vi "ContainsFile_WithFileIncluded_ReturnsTrue.vi"() -> ()   [LabVIEW 2019, in "WhitelistTest.lvlib"]
uses:
  WhitelistTest.lvlib
  Whitelist/Whitelist.lvclass
  Assertion/Assertion.lvlib
panel:
  out "error out":errorcluster
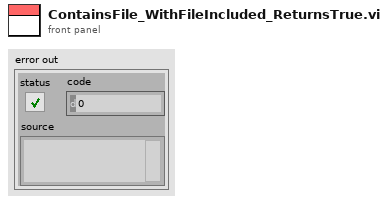
[diagram p1: front panel]
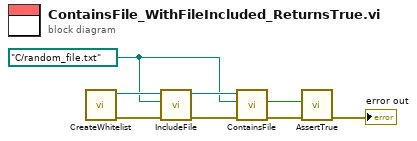
[diagram p0: block diagram]
diagram:
  w4 = path "C:/random_file.txt" ("Path")
  n1 = call "CreateWhitelist.vi"() -> ("error out"=w8:errorcluster, "Whitelist out"=w6:refnum<class "Whitelist.lvclass">)  [unwired: 10 in]
  n2 = call "IncludeFile.vi"("error in (no error)"=w8, "Path"=w4, "Whitelist in"=w6) -> ("error out"=w7:errorcluster, "Whitelist out"=w5:refnum<class "Whitelist.lvclass">)  [unwired: 7 in]
  n3 = call "ContainsFile.vi"("error in (no error)"=w7, "Path"=w4, "Whitelist in"=w5) -> ("error out"=w2:errorcluster, "Is Whitelisted?"=w3:bool)  [unwired: 6 in, 1 out]
  n4 = call "AssertTrue.vi"("error in (no error)"=w2, "Condition"=w3) -> ("error out"=→"error out":errorcluster)  [unwired: 9 in]
